vi "Comparison of mask2roi and label2roi.vi"() -> ()   [LabVIEW 2014]
uses:
  <vilib>/vision/NI_Vision_Development_Module.lvlib
panel:
  out "Src":T1(plugin-control)
  out "Mask2ROI after Label":T1(plugin-control)
  out "Label2ROI":T1(plugin-control)
  in  "Particle index":i32(slide) scale=0.0..5.0
  out "Mask2ROI":T1(plugin-control)
  # "Change  the index to see the particle overlayed.\n\nNote the output of Result of Label2Roi for index 0, it gives the background."
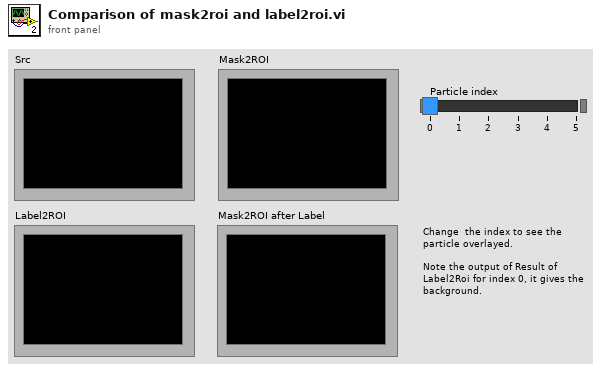
[diagram p1: front panel]
types:
  T1 = typedef "IMAQ Image.ctl" = refnum<image>
  T2 = typedef "ROI Descriptor" = cluster{"Global Rectangle":i32[], "Contours":cluster{"ID":enum32{"External", "Internal"}, "Type":u32, "Coordinates":i32[]}[]}
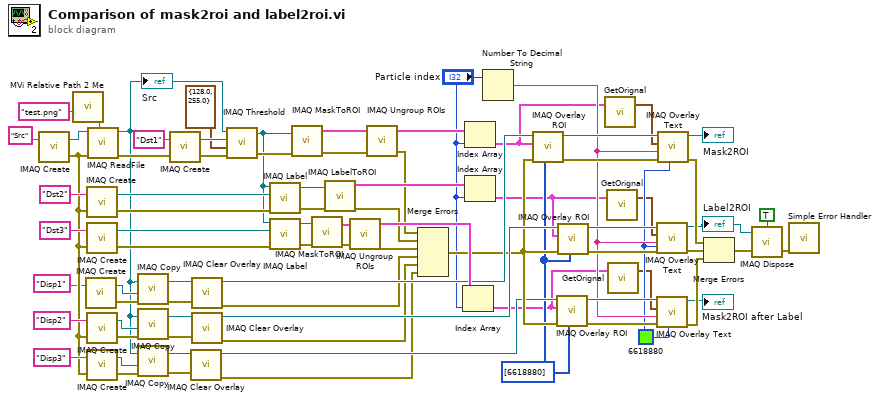
[diagram p0: block diagram]
diagram:
  w7 = u32 6618880 ("Text Color (black)")
  w25 = u32[] [6618880] ("Colors (Green)")
  n1 = call "IMAQ Create"("Image Name"="Src") -> ("New Image"=w70:T1, "error out"=w48:errorcluster)  [unwired: 4 in]
  n2 = call "MVi Relative Path 2 Me.vi"("Relative Path"="test.png") -> ("Appended Dir"=w42:path)  [unwired: 5 in, 1 out]
  n3 = call "IMAQ Create"("Image Name"="Disp1") -> ("New Image"=w39:T1, "error out"=w40:errorcluster)  [unwired: 4 in]
  n4 = call "IMAQ Create"("Image Name"="Dst2", "error in (no error)"=w48) -> ("New Image"=w66:T1, "error out"=w67:errorcluster)  [unwired: 3 in]
  n5 = call "IMAQ Create"("Image Name"="Dst3", "error in (no error)"=w48) -> ("New Image"=w60:T1, "error out"=w61:errorcluster)  [unwired: 3 in]
  n6 = call "IMAQ Create"("Image Name"="Disp2", "error in (no error)"=w48) -> ("New Image"=w52:T1, "error out"=w53:errorcluster)  [unwired: 3 in]
  n7 = call "IMAQ Create"("Image Name"="Disp3", "error in (no error)"=w48) -> ("New Image"=w51:T1, "error out"=w50:errorcluster)  [unwired: 3 in]
  n8 = call "IMAQ ReadFile"("File Path"=w42, "error in (no error)"=w48, "Image"=w70) -> ("error out"=w76:errorcluster, "Image Out"=w38:T1)  [unwired: 4 in, 3 out]
  "Src" <- w38
  n9 = call "IMAQ Copy"("error in (no error)"=w40, "Image Dst"=w39, "Image Src"=w38) -> ("error out"=w31:errorcluster, "Image Dst Out"=w37:T1)  [unwired: 3 in]
  n10 = call "IMAQ Copy"("error in (no error)"=w53, "Image Dst"=w52, "Image Src"=w38) -> ("error out"=w30:errorcluster, "Image Dst Out"=w36:T1)  [unwired: 3 in]
  n11 = call "IMAQ Copy"("error in (no error)"=w50, "Image Dst"=w51, "Image Src"=w38) -> ("error out"=w29:errorcluster, "Image Dst Out"=w33:T1)  [unwired: 3 in]
  n12 = call "IMAQ Create"("Image Name"="Dst1", "error in (no error)"=w76) -> ("New Image"=w79:T1, "error out"=w77:errorcluster)  [unwired: 3 in]
  n13 = call "IMAQ Clear Overlay"("error in (no error)"=w29, "Image"=w33) -> ("error out"=w26:errorcluster, "Image Out"=w32:T1)  [unwired: 8 in]
  n14 = call "IMAQ Clear Overlay"("error in (no error)"=w31, "Image"=w37) -> ("error out"=w28:errorcluster, "Image Out"=w63:T1)  [unwired: 8 in]
  n15 = call "IMAQ Clear Overlay"("error in (no error)"=w30, "Image"=w36) -> ("error out"=w27:errorcluster, "Image Out"=w35:T1)  [unwired: 8 in]
  n16 = call "IMAQ Threshold"("error in (no error)"=w77, "Range"=cluster{"Lower value":sgl, "Upper value":sgl} {"Lower value"=128.0, "Upper value"=255.0}, "Image Dst"=w79, "Image Src"=w38) -> ("error out"=w69:errorcluster, "Image Dst Out"=w59:T1)  [unwired: 6 in]
  n17 = call "IMAQ Label"("error in (no error)"=w67, "Image Dst"=w66, "Image Src"=w59) -> ("error out"=w65:errorcluster, "Image Dst Out"=w64:T1)  [unwired: 1 in, 1 out]
  n18 = call "IMAQ Label"("error in (no error)"=w61, "Image Dst"=w60, "Image Src"=w59) -> ("error out"=w58:errorcluster, "Image Dst Out"=w57:T1)  [unwired: 1 in, 1 out]
  n19 = call "IMAQ MaskToROI"("Image"=w59, "error in (no error)"=w69) -> ("ROI Descriptor"=w73:T2, "error out"=w74:errorcluster)  [unwired: 5 in, 1 out]
  n20 = call "IMAQ MaskToROI"("Image"=w57, "error in (no error)"=w58) -> ("ROI Descriptor"=w55:T2, "error out"=w56:errorcluster)  [unwired: 5 in, 1 out]
  n21 = call "IMAQ LabelToROI"("error in (no error)"=w65, "Image"=w64) -> ("error out"=w45:errorcluster, "ROIs"=w47:T2[])  [unwired: 6 in, 2 out]
  n22 = call "IMAQ Ungroup ROIs"("error in (no error)"=w56, "ROI Descriptor"=w55) -> ("error out"=w44:errorcluster, "ROI Descriptors out"=w80:T2[])  [unwired: 2 in]
  n23 = call "IMAQ Ungroup ROIs"("error in (no error)"=w74, "ROI Descriptor"=w73) -> ("error out"=w46:errorcluster, "ROI Descriptors out"=w75:T2[])  [unwired: 2 in]
  n24 = Merge Errors(w46, w45, w44, w28, w27, w26) -> (w34:errorcluster)
  n25 = Index Array(array=w80, index="Particle index") -> (element=w2:T2)
  n26 = Index Array(array=w75, index="Particle index") -> (element=w6:T2)
  n27 = Index Array(array=w47, index="Particle index") -> (element=w4:T2)
  n28 = Number To Decimal String(number="Particle index") -> (decimal integer string=w12:string)  [unwired: 1 in]
  n29 = call "IMAQ Overlay ROI"("Colors (Green)"=w25, "error in (no error)"=w34, "ROI Descriptor"=w6, "Image"=w63) -> ("error out"=w21:errorcluster, "Image Out"=w19:T1)  [unwired: 6 in]
  n30 = call "IMAQ Overlay ROI"("Colors (Green)"=w25, "error in (no error)"=w34, "ROI Descriptor"=w2, "Image"=w32) -> ("error out"=w14:errorcluster, "Image Out"=w13:T1)  [unwired: 6 in]
  n31 = call "IMAQ Overlay ROI"("Colors (Green)"=w25, "error in (no error)"=w34, "ROI Descriptor"=w4, "Image"=w35) -> ("error out"=w16:errorcluster, "Image Out"=w17:T1)  [unwired: 6 in]
  n32 = call "GetOrignal.vi"("element"=w6) -> ("Orignal"=w5:cluster{i32, i32})  [unwired: 2 in]
  n33 = call "GetOrignal.vi"("element"=w4) -> ("Orignal"=w3:cluster{i32, i32})  [unwired: 2 in]
  n34 = call "GetOrignal.vi"("element"=w2) -> ("Orignal"=w1:cluster{i32, i32})  [unwired: 2 in]
  n35 = call "IMAQ Overlay Text"("Text Color (black)"=w7, "error in (no error)"=w16, "String"=w12, "Origin"=w3, "Image"=w17) -> ("error out"=w15:errorcluster, "Image Out"=w8:T1)  [unwired: 5 in]
  "Label2ROI" <- w8
  n36 = call "IMAQ Overlay Text"("Text Color (black)"=w7, "error in (no error)"=w14, "String"=w12, "Origin"=w1, "Image"=w13) -> ("error out"=w11:errorcluster, "Image Out"=→"Mask2ROI after Label":T1)  [unwired: 5 in]
  n37 = call "IMAQ Overlay Text"("Text Color (black)"=w7, "error in (no error)"=w21, "String"=w12, "Origin"=w5, "Image"=w19) -> ("error out"=w18:errorcluster, "Image Out"=→"Mask2ROI":T1)  [unwired: 5 in]
  n38 = Merge Errors(w18, w15, w11) -> (w24:errorcluster)
  n39 = call "IMAQ Dispose"("All Images? (No)"=TRUE, "Image"=w8, "error in (no error)"=w24) -> ("error out"=w22:errorcluster)  [unwired: 3 in]
  n40 = call <vilib>:"Simple Error Handler.vi"("error in (no error)"=w22) -> ()  [unwired: 4 in, 5 out]
